vi "Initialize RxTx.vi"(8 "error in (no error)":errorcluster, 11 "Filter_Wheel in":refnum<class "Filter_Wheel.lvclass">) -> (0 "error out":errorcluster, 3 "Filter_Wheel out":refnum<class "Filter_Wheel.lvclass">)   [LabVIEW 2018, in "Filter_Wheel.lvclass"]
uses:
  Filter_Wheel.lvclass
  Filter_Wheel.lvclass/Filter_Wheel.ctl
  RxTx/RxTx.lvclass
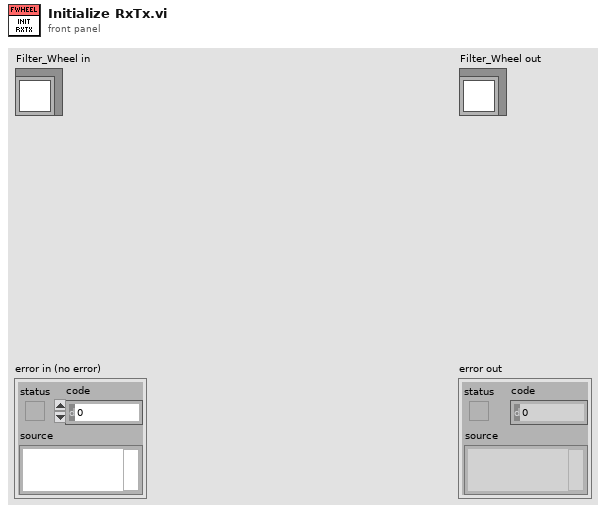
[diagram p1: front panel]
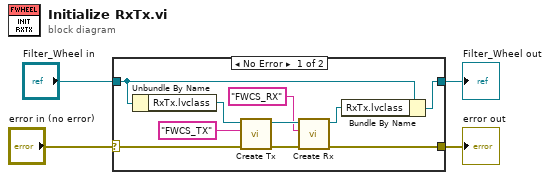
[diagram p0: block diagram]
diagram:
  n1 = case shown="No Error" "error in (no error)" {
    selector: "error in (no error)" -> [w12 w16]
    tunnel: [w10 w16] -> w3
    tunnel: [w13 w15] -> w1
    tunnel: "Filter_Wheel in" -> [w14 w15]
    frame No Error {
      n2 = Unbundle By Name(w14) -> ("RxTx.lvclass"=w7:refnum<class "RxTx.lvclass">)
      n3 = call "Create Tx.vi"("error in (no error)"=w12, "Writer Name"="FWCS_TX", "RxTx in"=w7) -> ("error out"=w11:errorcluster, "RxTx out"=w8:refnum<class "RxTx.lvclass">)  [unwired: 7 in]
      n4 = call "Create Rx.vi"("error in (no error)"=w11, "Reader Name"="FWCS_RX" ("Writer Name"), "RxTx in"=w8) -> ("error out"=w10:errorcluster, "RxTx out"=w9:refnum<class "RxTx.lvclass">)  [unwired: 7 in]
      n5 = Bundle By Name(cluster=w14, "RxTx.lvclass"=w9) -> (w13:refnum<class "Filter_Wheel.lvclass">)
    }
    frame Error {
    }
  }
  "error out" <- w3
  "Filter_Wheel out" <- w1
